vi "PID Elbow Range.vi"(1 "Input PID":dbl) -> (0 "Output Range":dbl)   [LabVIEW 2017]
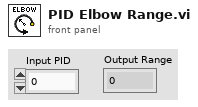
[diagram p1: front panel]
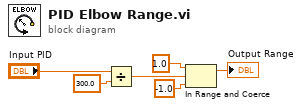
[diagram p0: block diagram]
diagram:
  n1 = Divide(x="Input PID", y=300.0) -> (x/y=w3:dbl)
  n2 = In Range and Coerce(upper limit=1.0, x=w3, lower limit=-1.0) -> (coerced(x)=→"Output Range":dbl)  [unwired: 1 out]
